vi "Queue In Array.vi"(7 "First":bool, 8 "error in (no error)":errorcluster caption="Error In", 9 "Data":variant[](array[variant]), 10 "Message":string[](array[string]), 11 "Queue In":refnum<queue>) -> (0 "error out":errorcluster caption="Error Out", 3 "Queue Out":refnum<queue>)   [LabVIEW 2020]
uses:
  Queue Message.ctl
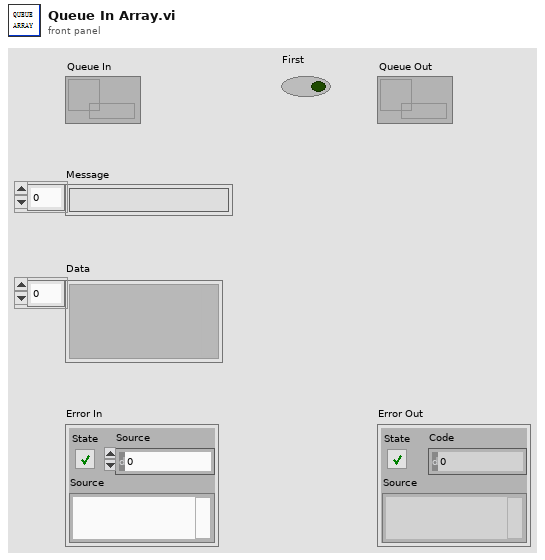
[diagram p1: front panel]
types:
  T1 = typedef "Queue Message.ctl" = cluster{"Message":string, "Data":variant}
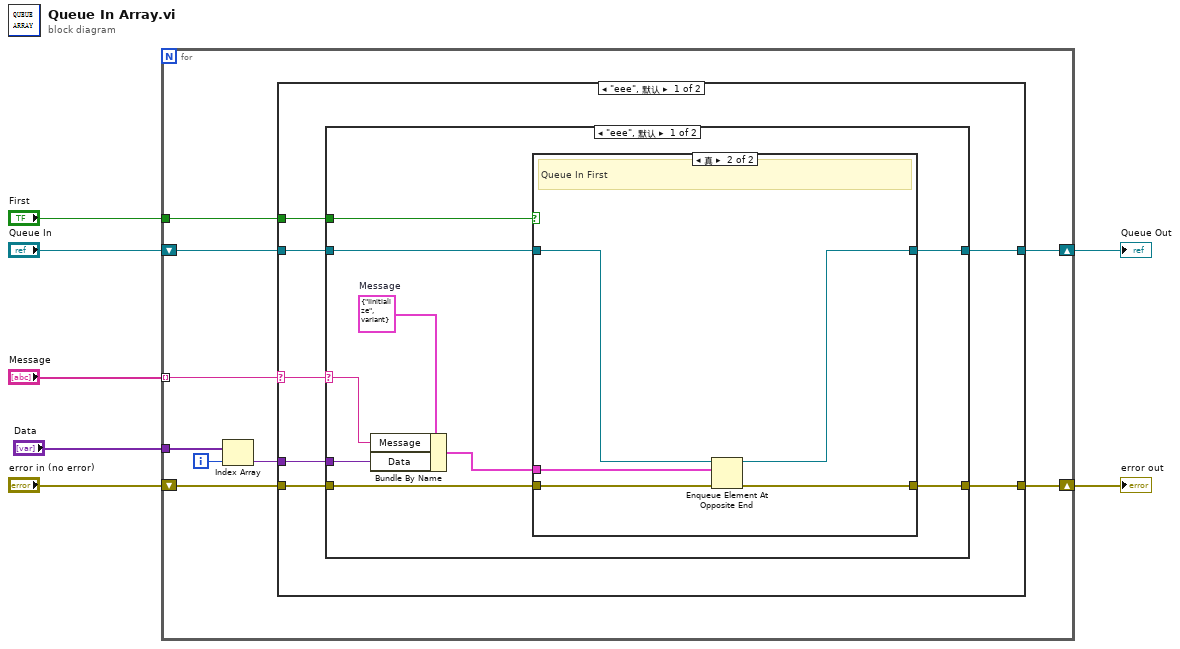
[diagram p0: block diagram]
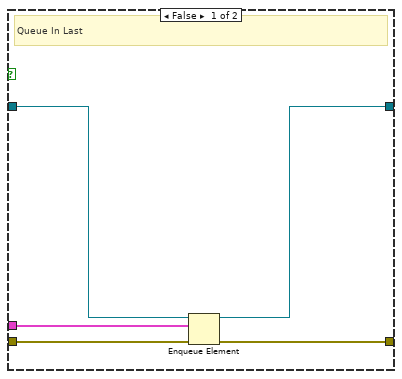
[diagram p2: hidden frame]
diagram:
  n1 = for {
    tunnel: "Data" -> [w10]
    tunnel: "First" -> [w12]
    tunnel: "Message" -> [w11] mode=indexing
    shift-right: [w15] -> w6
    shift-left: "Queue In" -> [w16]
    shift-right: [w13] -> w3
    shift-left: "error in (no error)" -> [w14]
    i -> [w9]
    n2 = Index Array(array=w10, index=w9) -> (element=w8:variant)
    n3 = case shown="\"eee\", 默认" w11 {
      selector: w11 -> [w17 _]
      tunnel: w16 -> [w23 w45]
      tunnel: [w22 w45] -> w15
      tunnel: w8 -> [w21 _]
      tunnel: w14 -> [w20 w46]
      tunnel: [w19 w46] -> w13
      tunnel: w12 -> [w18 _]
      frame "eee", Default {
        n4 = case shown="\"eee\", 默认" w17 {
          selector: w17 -> [w25 _]
          tunnel: w23 -> [w32 w44]
          tunnel: [w31 w44] -> w22
          tunnel: w21 -> [w29 _]
          tunnel: w20 -> [w28 w43]
          tunnel: [w27 w43] -> w19
          tunnel: w18 -> [w26 _]
          frame "eee", Default {
            w24 = T1 {"Message"="Iinitialize", "Data"=variant}  # Message
            n5 = Bundle By Name(cluster=w24, "Message"=w25, "Data"=w29) -> (w30:T1)
            n6 = case shown="真" w26 {
              tunnel: w32 -> [w37 w42]
              tunnel: [w36 w39] -> w31
              tunnel: w30 -> [w35 w38]
              tunnel: w28 -> [w34 w41]
              tunnel: [w33 w40] -> w27
              frame False {
                # "Queue In Last"
                n7 = Enqueue Element(queue=w37, element=w35, error in (no error)=w34) -> (queue out=w36:refnum<queue>, error out=w33:errorcluster)  [unwired: 1 in, 1 out]
              }
              frame True {
                # "Queue In First"
                n8 = Enqueue Element At Opposite End(queue=w42, element=w38, error in (no error)=w41) -> (queue out=w39:refnum<queue>, error out=w40:errorcluster)  [unwired: 1 in, 1 out]
              }
            }
          }
          frame "" {
          }
        }
      }
      frame "" {
      }
    }
  }
  "Queue Out" <- w6
  "error out" <- w3
